vi "Autonomous Independent_OLD.vi"   [LabVIEW 2013]
uses:
  <vilib>/Rock Robotics/WPI/Solenoid/WPI_SolenoidValue.ctl
  <vilib>/Rock Robotics/WPI/RobotDrive/WPI_RobotDriveGetSetRefNum.vi
  <vilib>/Rock Robotics/WPI/Solenoid/WPI_SolenoidSetEnum.vi
  <vilib>/Rock Robotics/WPI/RobotDrive/WPI_RobotDriveArcadeDrive_Standard(NoSaturation).vi
types:
  T1 = typedef "WPI_MotorControlDeviceRef.ctl" = cluster{"DeviceStatus":errorcluster, "Type":enum16{"PWM", "CAN"}, "PWM":cluster{"Digital Module":T2, "PWM Channel":T3, "DeadBand":T4}, "CAN":cluster{"Device Number":u8, "Control Mode":T5, "Semaphore":T6, "Max Vout":dbl}, "Invert":bool, "TransformRef":T7, "InvTransformRef":T7}
  T2 = typedef "FPGA_TypedefDigitalModule.ctl" = enum16{"Digital Module 1", "Digital Module 2"}
  T3 = typedef "FPGA_DIOPWMChannel.ctl" = enum8{"PWM 1", "PWM 2", "PWM 3", "PWM 4", "PWM 5", "PWM 6", "PWM 7", "PWM 8", "PWM 9", "PWM 10", "Invalid"}
  T4 = typedef "WPI_PWMDeadband.ctl" = cluster{"Name":string, "maxPositivePwm":i32, "minPositivePwm":i32, "centerPwm":i32, "maxNegativePwm":i32, "minNegativePwm":i32, "angularRange":u16}
  T5 = typedef "WPI_CANJaguar_ControlMode.ctl" = enum8{"Percent VBus", "Current", "Speed", "Position", "Voltage"}
  T6 = typedef "Semaphore RefNum" = refnum<k1>
  T7 = typedef "WPI_PWMTransform_ConPane.ctl" = refnum<vi>
  T8 = typedef "WPI_SolenoidDevRef.ctl" = cluster{"DevStatus":errorcluster, "Solenoid Module":T9, "Forward Solenoid Channel":T10, "Reverse Solenoid Channel":T10}
  T9 = typedef "FPGA_TypedefSolenoidModule.ctl" = enum16{"Solenoid Module 1", "Solenoid Module 2"}
  T10 = typedef "WPI_SolenoidChannel.ctl" = enum8{"Solenoid 1", "Solenoid 2", "Solenoid 3", "Solenoid 4", "Solenoid 5", "Solenoid 6", "Solenoid 7", "Solenoid 8", "Invalid"}
  T11 = typedef "WPI_DigitalInputDevRef.ctl" = cluster{"DevStatus":errorcluster, "DIO Channel":T12, "Digital Module":T2}
  T12 = typedef "FPGA_DIOChannel.ctl" = enum8{"DIO 1", "DIO 2", "DIO 3", "DIO 4", "DIO 5", "DIO 6", "DIO 7", "DIO 8", "DIO 9", "DIO 10", "DIO 11", "DIO 12", "DIO 13", "DIO 14", "Invalid"}
  T13 = typedef "WPI_RobotDriveDevRef.ctl" = cluster{"DevStatus":errorcluster, "Motors[]":T1[], "Square Inputs":bool, "Max Output":dbl, "Isochronous":bool}
  T14 = typedef "WPI_SolenoidValue.ctl" = enum16{"Off", "On", "Forward", "Reverse"}
  T15 = typedef "WPI_UltrasonicDeviceRef.ctl" = cluster{"DevStatus":errorcluster, "Ping Digital Module":T2, "Echo Digital Module":T2, "Ping Channel":T12, "Echo Channel":T12, "CntIndex":T16}
  T16 = typedef "FPGA_CounterCtrSystemIndex.ctl" = enum8{"Ctr 0", "Ctr 1", "Ctr 2", "Ctr 3", "Ctr 4", "Ctr 5", "Ctr 6", "Ctr 7", "Invalid"}
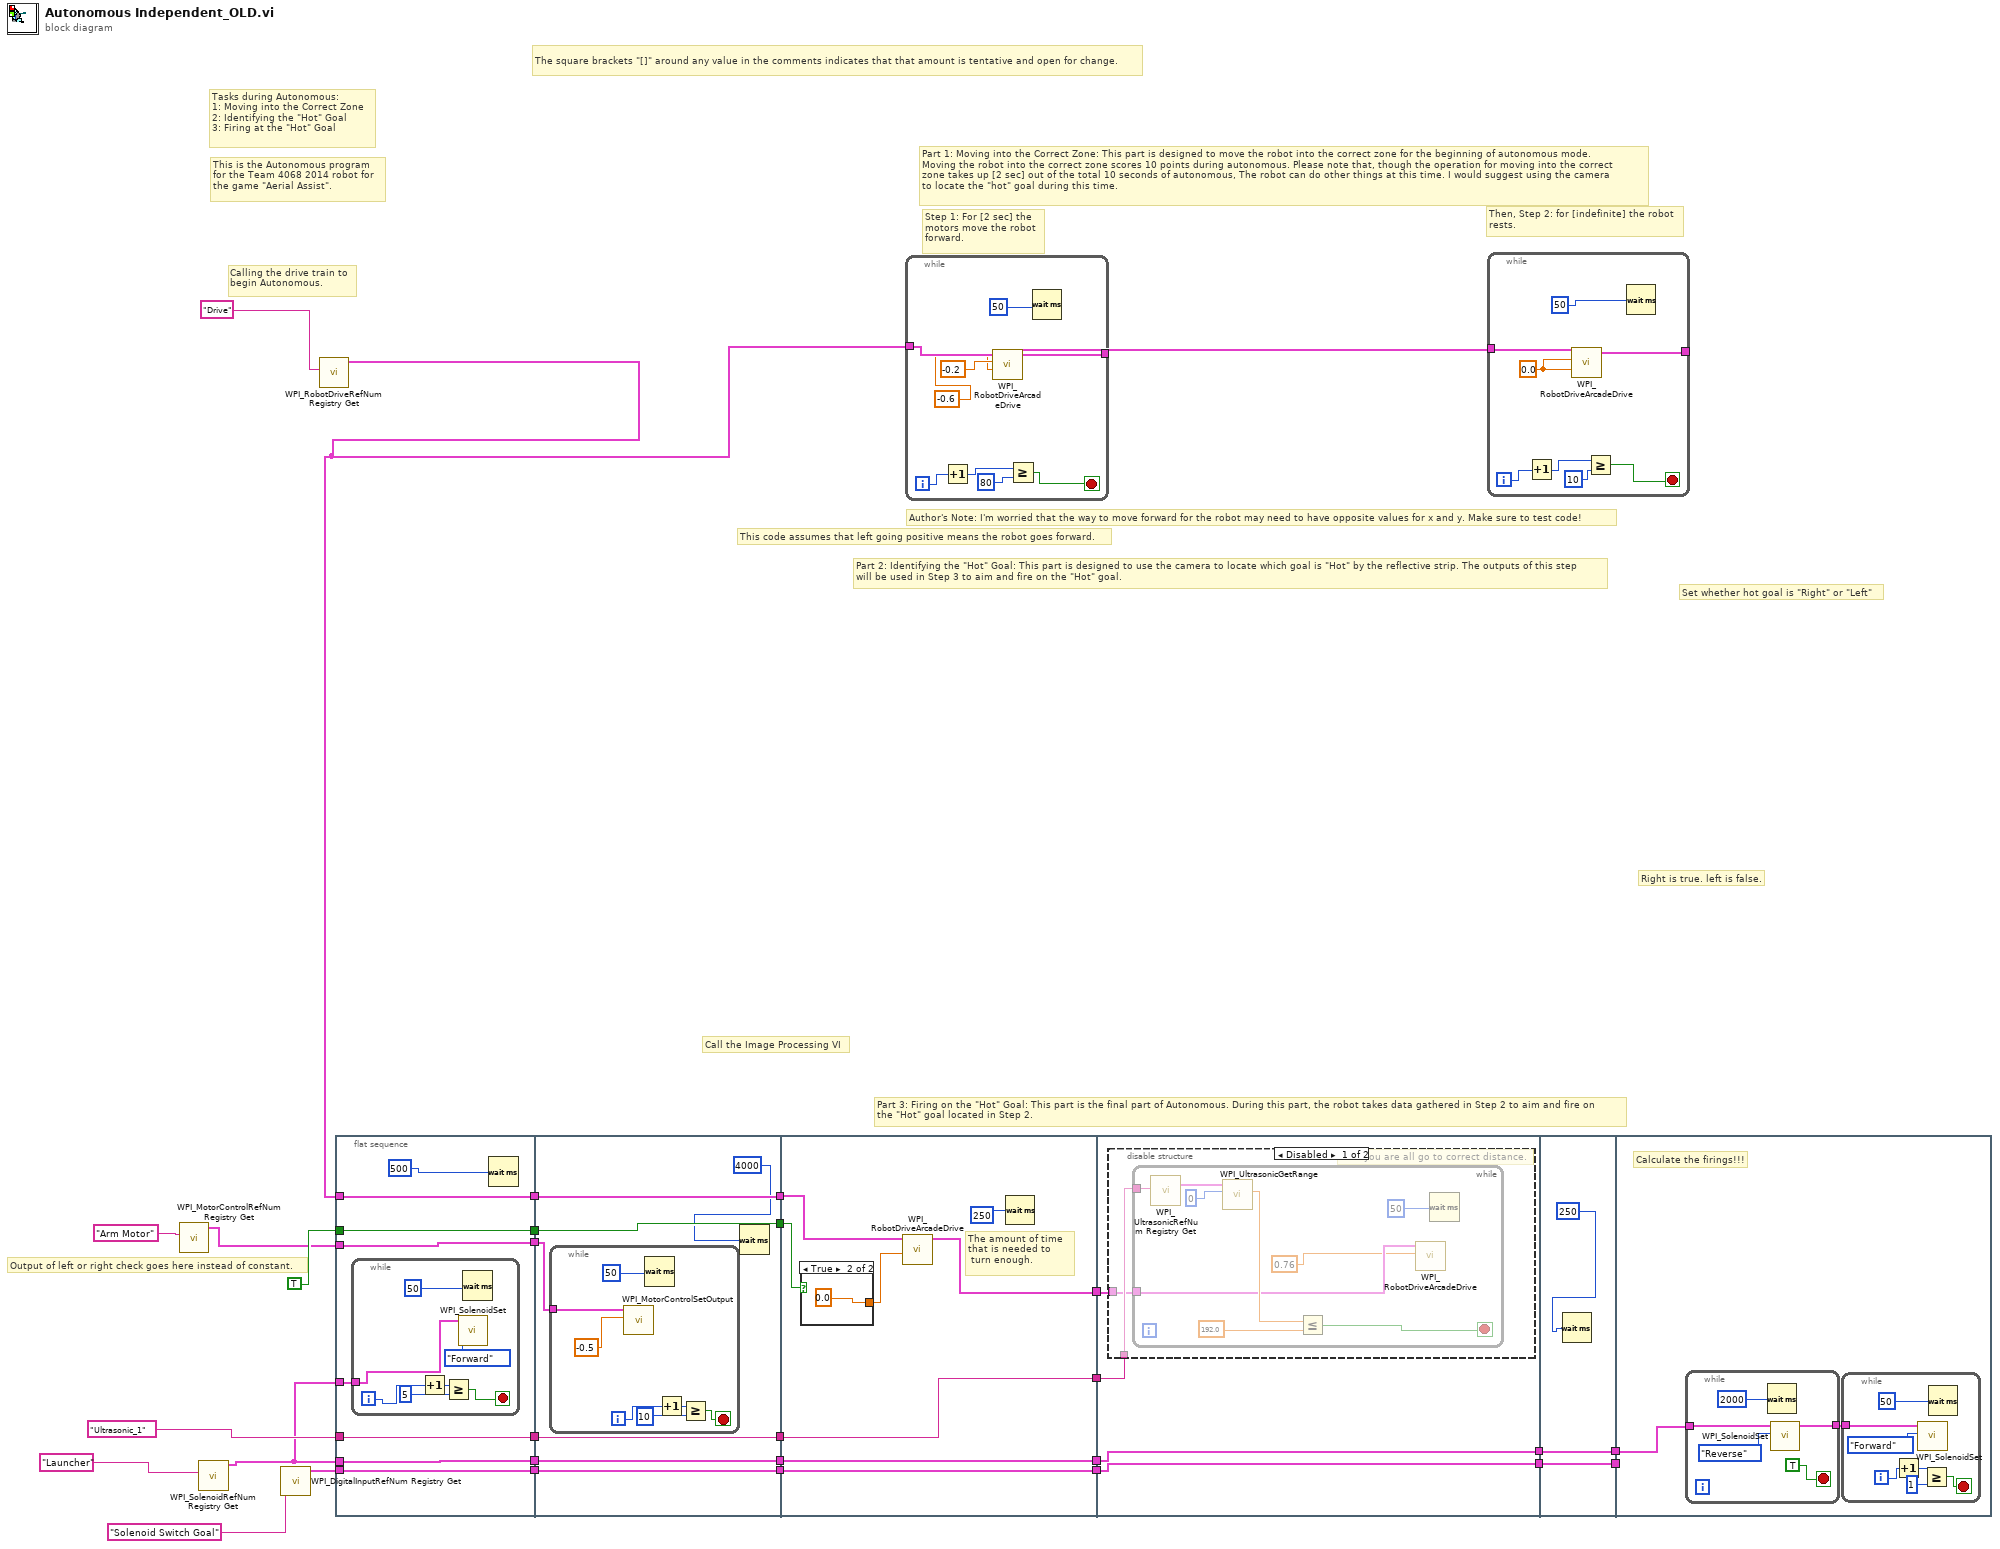
[diagram p0: block diagram]
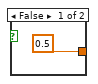
[diagram p2: hidden frame]
diagram:
  # "Output of left or right check goes here instead of constant."
  # "Call the Image Processing VI"
  # "Part 3: Firing on the \"Hot\" Goal: This part is the final part of Autonomous. During this part, the robot takes data gathered in Step 2 to aim and fire on \nthe \"Hot\" goal located in Step 2."
  # "Right is true. left is false."
  # "Set whether hot goal is \"Right\" or \"Left\""
  # "Part 2: Identifying the \"Hot\" Goal: This part is designed to use the camera to locate which goal is \"Hot\" by the reflective strip. The outputs of this step\nwill be used in Step 3 to aim and fire on the \"Hot\" goal."
  # "Tasks during Autonomous:\n1: Moving into the Correct Zone\n2: Identifying the \"Hot\" Goal\n3: Firing at the \"Hot\" Goal"
  # "This code assumes that left going positive means the robot goes forward."
  # "Author's Note: I'm worried that the way to move forward for the robot may need to have opposite values for x and y. Make sure to test code!"
  # "Part 1: Moving into the Correct Zone: This part is designed to move the robot into the correct zone for the beginning of autonomous mode.\nMoving the robot into the correct zone scores 10 points during autonomous. Please note that, though the operation for moving into the correct\nzone takes up [2 sec] out of the total 10 seconds of autonomous, The robot can do other things at this time. I would suggest using the camera \nto locate the \"hot\" goal during this time."
  # "The square brackets \"[]\" around any value in the comments indicates that that amount is tentative and open for change."
  # "This is the Autonomous program \nfor the Team 4068 2014 robot for \nthe game \"Aerial Assist\"."
  # "Then, Step 2: for [indefinite] the robot \nrests."
  # "Step 1: For [2 sec] the \nmotors move the robot\nforward."
  # "Calling the drive train to \nbegin Autonomous."
  n1 = call <vilib>:"WPI_MotorControlRefNum Registry Get.vi"("refnum name"="Arm Motor") -> ("MotorControlDevRef"=w4:T1)  [unwired: 9 in, 1 out]
  n2 = call <vilib>:"WPI_SolenoidRefNum Registry Get.vi"("refnum name"="Launcher") -> ("SolenoidDevRef"=w1:T8)  [unwired: 9 in, 1 out]
  n3 = call <vilib>:"WPI_DigitalInputRefNum Registry Get.vi"("refnum name"="Solenoid Switch Goal") -> ("DigitalInputDevRef"=w6:T11)  [unwired: 9 in, 1 out]
  n4 = call <vilib>:"WPI_RobotDriveRefNum Registry Get.vi"("refnum name"="Drive") -> ("RobotDriveDevRef"=w28:T13)  [unwired: 9 in, 1 out]
  n5 = flat-sequence {
    tunnel: w4 -> [w34]
    tunnel: w6 -> [w35]
    tunnel: TRUE -> [w36]
    tunnel: "Ultrasonic_1" -> [w37]
    tunnel: w28 -> [w38]
    tunnel: [w38] -> w27
    tunnel: [w37] -> w26
    tunnel: [w36] -> w25
    tunnel: [w35] -> w24
    tunnel: [w34] -> w23
    tunnel: w1 -> [w32]
    tunnel: [w31] -> w22
    tunnel: w1 -> [w31]
    tunnel: [w52] -> w21
    tunnel: [w51] -> w20
    tunnel: [w50] -> w19
    tunnel: [w49] -> w18
    tunnel: w27 -> [w52]
    tunnel: w26 -> [w51]
    tunnel: w25 -> [w50]
    tunnel: w24 -> [w49]
    tunnel: w23 -> [w47]
    tunnel: w22 -> [w46]
    tunnel: [w46] -> w17
    tunnel: [w65] -> w16
    tunnel: [w62] -> w15
    tunnel: [w61] -> w14
    tunnel: w21 -> [w67]
    tunnel: w20 -> [w65]
    tunnel: w19 -> [w63]
    tunnel: w18 -> [w61]
    tunnel: [w60] -> w13
    tunnel: w17 -> [w60]
    tunnel: w16 -> [w73]
    tunnel: w15 -> [w72]
    tunnel: w14 -> [w71]
    tunnel: [w71] -> w12
    tunnel: w13 -> [w70]
    tunnel: [w70] -> w11
    tunnel: [w86] -> w10
    tunnel: w12 -> [w86]
    tunnel: [w85] -> w9
    tunnel: w11 -> [w85]
    tunnel: w10 -> [_]
    tunnel: w9 -> [w88]
    frame #0 {
      n6 = while {
        tunnel: w32 -> [w40]
        i -> [w42]
        stop <- w41 stop-if-true
        n7 = Increment(x=w42) -> (x+1=w44:i32)
        n8 = Greater Or Equal?(x=w44, y=5) -> (x >= y?=w41:bool)
        n9 = call-poly <vilib>:"WPI_SolenoidSet.vi"("Value"=WPI_SolenoidValue."Forward", "SolenoidDevRef"=w40) -> ()  [unwired: 8 in, 2 out]
        n10 = Wait (ms)(milliseconds to wait=50) -> ()  [unwired: 1 out]
      }
      n11 = Wait (ms)(milliseconds to wait=500) -> ()  [unwired: 1 out]
    }
    frame #1 {
      n12 = while {
        tunnel: w47 -> [w54]
        i -> [w59]
        stop <- w56 stop-if-true
        n13 = call <vilib>:"WPI_MotorControlSetOutput.vi"("Output"=-0.5, "MotorControlDevRef"=w54) -> ()  [unwired: 7 in, 3 out]
        n14 = Wait (ms)(milliseconds to wait=50) -> ()  [unwired: 1 out]
        n15 = Increment(x=w59) -> (x+1=w58:i32)
        n16 = Greater Or Equal?(x=w58, y=10) -> (x >= y?=w56:bool)
      }
      n17 = Wait (ms)(milliseconds to wait=4000) -> ()  [unwired: 1 out]
    }
    frame #2 {
      # "The amount of time \nthat is needed to\n turn enough."
      n18 = case shown="True" w63 {
        tunnel: [0.5 0.0] -> w64
        frame False {
        }
        frame True {
        }
      }
      n19 = call-poly <vilib>:"WPI_RobotDriveArcadeDrive.vi"("Y axis value"=w64, "RobotDriveDevRef"=w67) -> ("RobotDriveDevRef"=w62:T13)  [unwired: 7 in, 2 out]
      n20 = Wait (ms)(milliseconds to wait=250) -> ()  [unwired: 1 out]
    }
    frame #3 {
      n21 = disable-structure shown="Disabled" {
        disable-tunnel: w73 -> [w75 _]
        disable-tunnel: w72 -> [w74 _]
        frame Disabled {
          # "First you are all go to correct distance."
          n22 = while {
            tunnel: w75 -> [w84]
            tunnel: w74 -> [w78]
            stop <- w80 stop-if-true
            n23 = call <vilib>:"WPI_UltrasonicRefNum Registry Get.vi"("refnum name"=w84) -> ("UltrasonicDevRef"=w83:T15)  [unwired: 9 in, 1 out]
            n24 = call <vilib>:"WPI_UltrasonicGetRange.vi"("Range Units"=0, "UltrasonicDevRef"=w83) -> ("Distance"=w81:dbl)  [unwired: 7 in, 2 out]
            n25 = Less Or Equal?(x=w81, y=192.0) -> (x <= y?=w80:bool)
            n26 = call-poly <vilib>:"WPI_RobotDriveArcadeDrive.vi"("X axis value"=0.76, "RobotDriveDevRef"=w78) -> ()  [unwired: 7 in, 3 out]
            n27 = Wait (ms)(milliseconds to wait=50) -> ()  [unwired: 1 out]
          }
        }
        frame Enabled {
        }
      }
    }
    frame #4 {
      n28 = Wait (ms)(milliseconds to wait=250) -> ()  [unwired: 1 out]
    }
    frame #5 {
      # "Calculate the firings!!!"
      n29 = while {
        tunnel: w88 -> [w101]
        tunnel: [w100] -> w89
        stop <- TRUE stop-if-true
        n30 = Wait (ms)(milliseconds to wait=2000) -> ()  [unwired: 1 out]
        n31 = call-poly <vilib>:"WPI_SolenoidSet.vi"("Value"=WPI_SolenoidValue."Reverse", "SolenoidDevRef"=w101) -> ("SolenoidDevRef"=w100:T8)  [unwired: 8 in, 1 out]
      }
      n32 = while {
        tunnel: w89 -> [w96]
        i -> [w94]
        stop <- w91 stop-if-true
        n33 = Increment(x=w94) -> (x+1=w93:i32)
        n34 = call-poly <vilib>:"WPI_SolenoidSet.vi"("Value"=WPI_SolenoidValue."Forward", "SolenoidDevRef"=w96) -> ()  [unwired: 8 in, 2 out]
        n35 = Greater Or Equal?(x=w93, y=1) -> (x >= y?=w91:bool)
        n36 = Wait (ms)(milliseconds to wait=50) -> ()  [unwired: 1 out]
      }
    }
  }
  n37 = while {
    tunnel: w28 -> [w110]
    tunnel: [w109] -> w29
    i -> [w108]
    stop <- w105 stop-if-true
    n38 = Increment(x=w108) -> (x+1=w107:i32)
    n39 = call-poly <vilib>:"WPI_RobotDriveArcadeDrive.vi"("Y axis value"=-0.6, "X axis value"=-0.2, "RobotDriveDevRef"=w110) -> ("RobotDriveDevRef"=w109:T13)  [unwired: 6 in, 2 out]
    n40 = Greater Or Equal?(x=w107, y=80) -> (x >= y?=w105:bool)
    n41 = Wait (ms)(milliseconds to wait=50) -> ()  [unwired: 1 out]
  }
  n42 = while {
    tunnel: w29 -> [w118]
    tunnel: [w116] -> _
    i -> [w114]
    stop <- w111 stop-if-true
    w117 = 0.0
    n43 = Increment(x=w114) -> (x+1=w112:i32)
    n44 = call-poly <vilib>:"WPI_RobotDriveArcadeDrive.vi"("Y axis value"=w117, "X axis value"=w117, "RobotDriveDevRef"=w118) -> ("RobotDriveDevRef"=w116:T13)  [unwired: 6 in, 2 out]
    n45 = Greater Or Equal?(x=w112, y=10) -> (x >= y?=w111:bool)
    n46 = Wait (ms)(milliseconds to wait=50) -> ()  [unwired: 1 out]
  }
